vi "time.vi"(8 "error in (no error)":errorcluster caption="错误输入（无错误）", 9 "END":u32, 11 "START":u32) -> (0 "error out":errorcluster caption="错误输出", 2 "Elapsed Time Text":string caption="Elapsed Time")   [LabVIEW 2018]
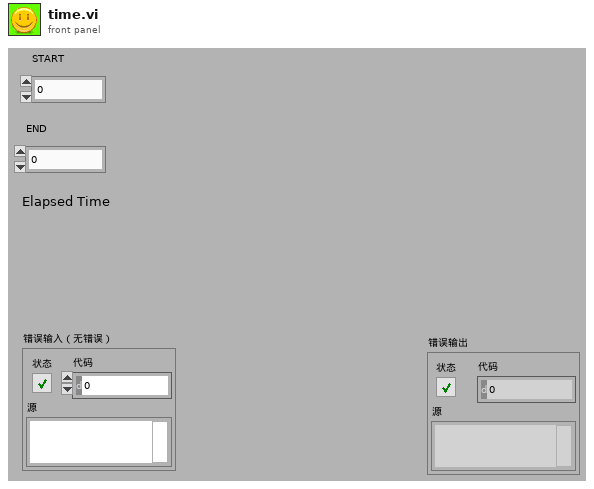
[diagram p1: front panel]
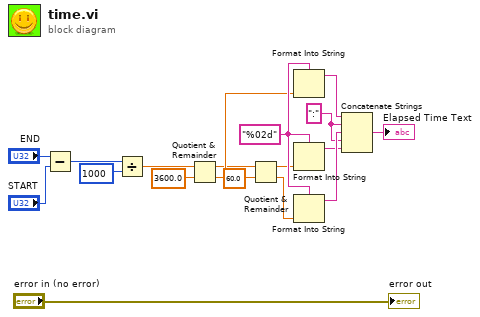
[diagram p0: block diagram]
diagram:
  w16 = "%02d" ("格式字符串")
  w11 = ":"
  n1 = Subtract(x="END", y="START") -> (x-y=w8:u32)
  n2 = Divide(x=w8, y=u32 1000) -> (x/y=w6:dbl)
  n3 = Quotient & Remainder(x=w6, y=3600.0) -> (x-y*floor(x/y)=w4:dbl, floor(x/y)=w5:dbl)
  n4 = Quotient & Remainder(x=w4, y=60.0) -> (x-y*floor(x/y)=w13:dbl, floor(x/y)=w15:dbl)
  n5 = Format Into String(format string=w16, w5) -> (resulting string=w17:string)  [unwired: 2 in, 1 out]
  n6 = Format Into String(format string=w16, w13) -> (resulting string=w14:string)  [unwired: 2 in, 1 out]
  n7 = Format Into String(format string=w16, w15) -> (resulting string=w18:string)  [unwired: 2 in, 1 out]
  n8 = Concatenate Strings(w17, w11, w18, w11, w14) -> (→"Elapsed Time Text":string)
  "error out" <- "error in (no error)"
